vi "Main.vi"() -> ()   [LabVIEW 2024]
doc: "This template is for the Queued Message Handler design pattern.\n\nThe Event Handling Loop generates messages based on user interface actions.\n\nThe Message Handling Loop processes messages generated by the Event Handling Loop, or by other messages. The messages are string values, so new messages can be added easily to the Message Cases case structure in the Message Handling Loop. Each message cluster can also provide an optional value for Message Data, which is a variant that can be converted to whatever message-specific data is required."
uses:
  controls/UI Data.ctl
  support/Message Queue/Enqueue Message (Single).vi
  <vilib>/Utility/error.llb/Error Cluster From Error Code.vi
  <vilib>/ErrorRing/Error Ring.xnode
  support/Message Queue/Message Queue.lvlib
  support/User Event - Stop/User Event - Stop.lvlib
panel:
  out "Display <Replace Me>":string
  in  "Do Something Else <Replace Me>":bool
  in  "Do Something <Replace Me>":bool
  in  "Exit":bool
  # "These controls have associated \"Value Changed\" events configured in the Event Structure on the diagram.\n\nReplace them (and reconfigure the Event Structure) with the controls you need for your application."
  # "This template is for the Queued Message Handler design pattern.\n\nSee the block diagram for more information on how to use this template."
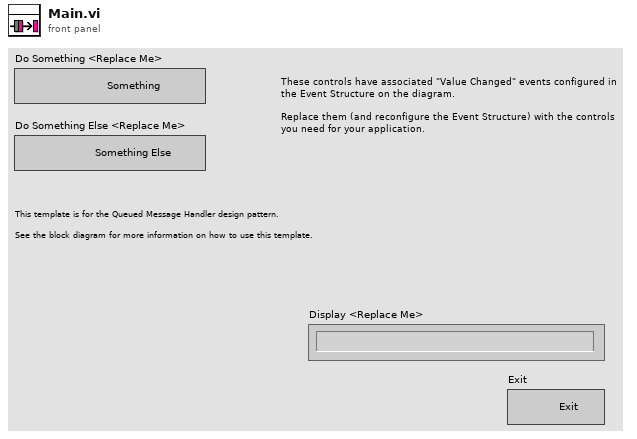
[diagram p1: front panel]
types:
  T1 = typedef "UI Data.ctl" = cluster{"Boolean <Replace Me>":bool, "String <Replace Me>":string, "Numeric <Replace Me>":dbl, "ADK Create MT":refnum<vi>, "ADK Stop":refnum<vi>, "Data Display Ref":refnum<vi>, "Exit Button Ref":refnum<vi>, " ADK Close":refnum<vi>}
  T2 = typedef "Message Queue.lvlib/All Message Queues.ctl" = cluster{"UI":refnum<queue>}
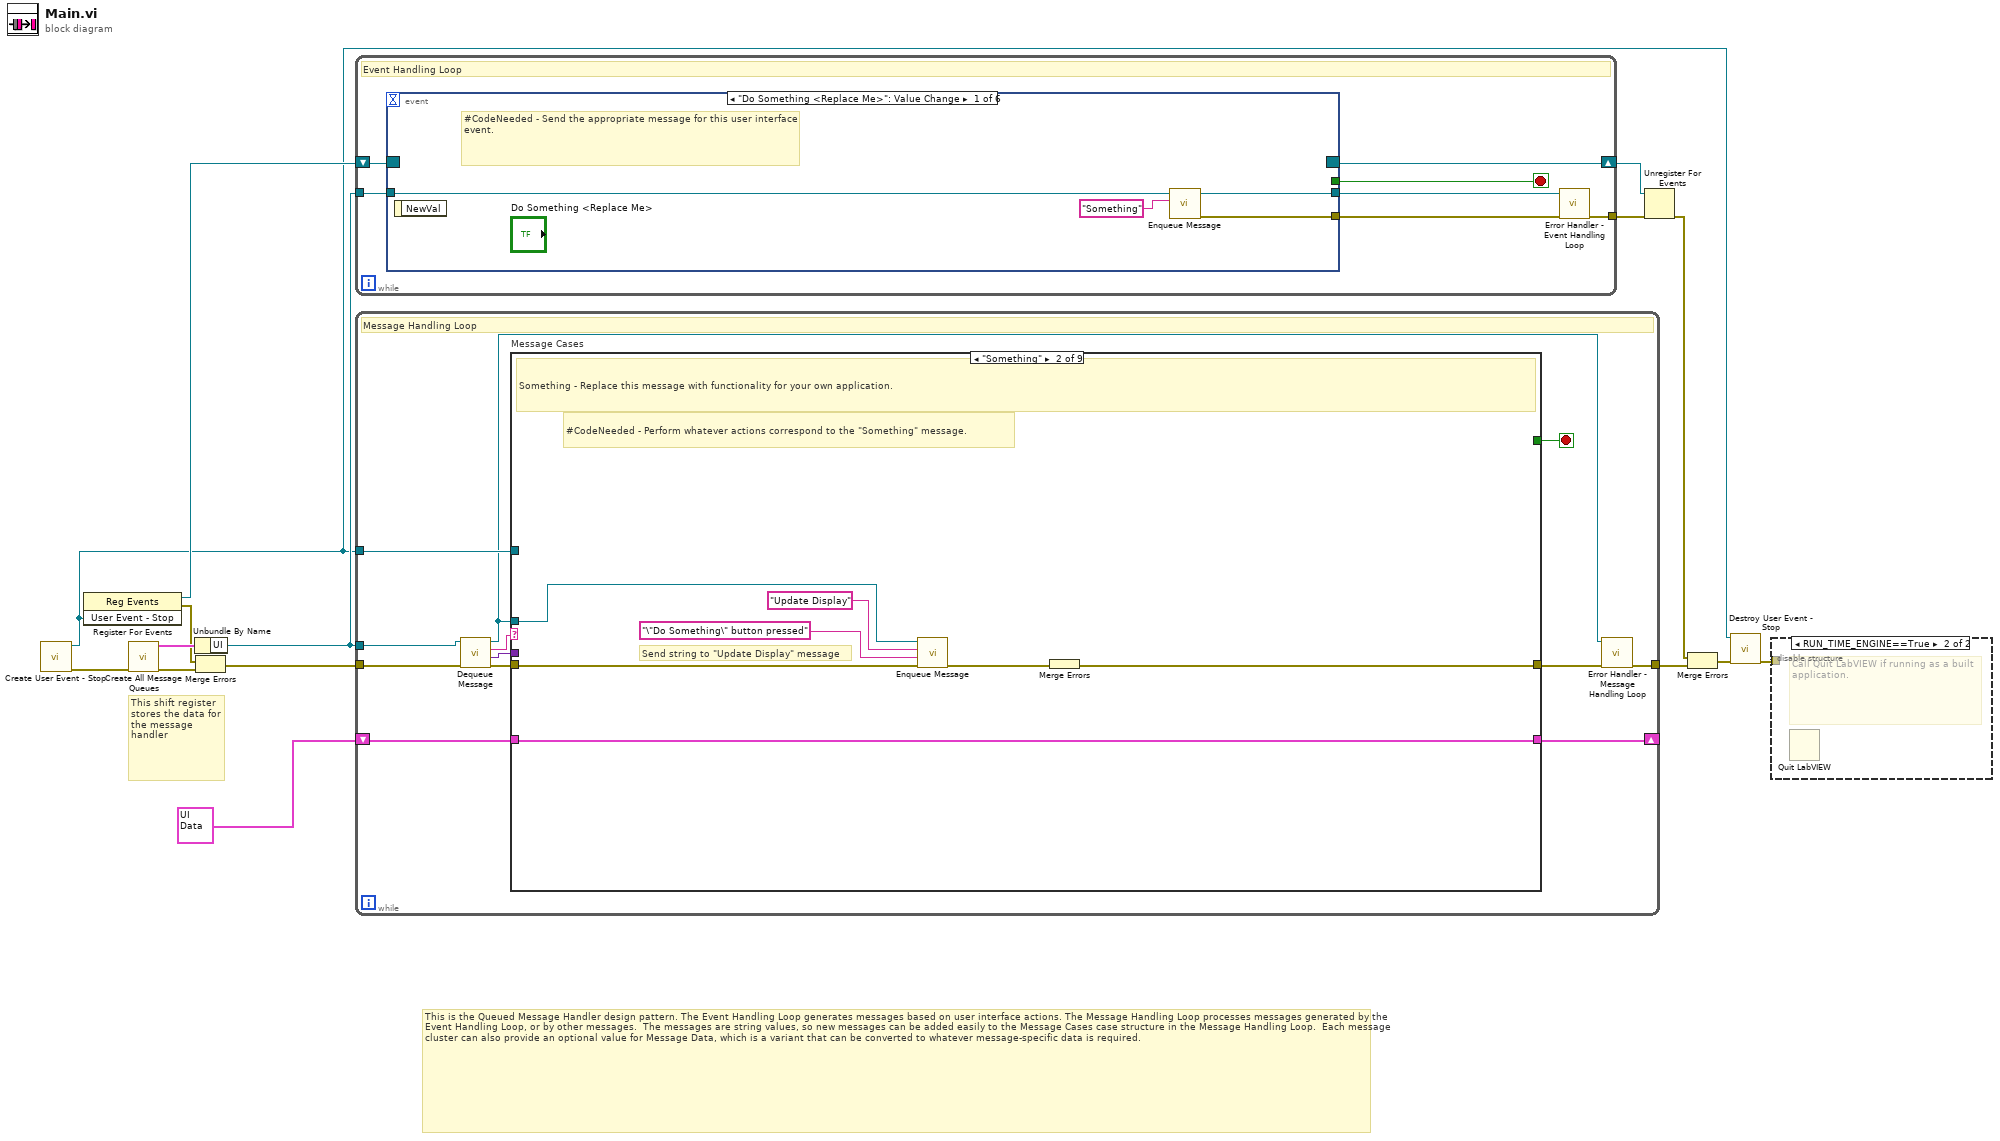
[diagram p0: block diagram]
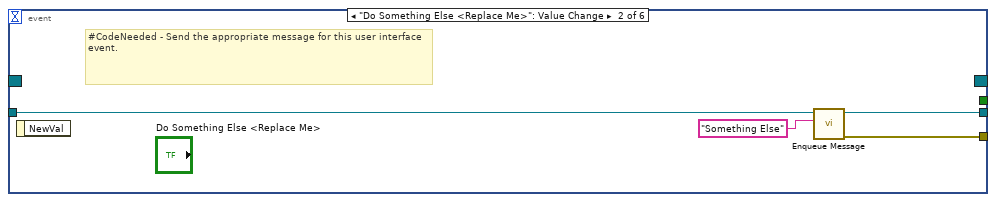
[diagram p3: hidden frame]
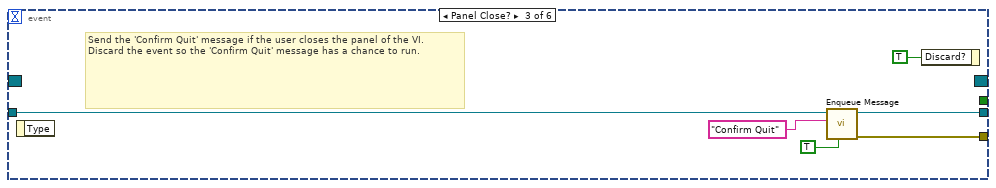
[diagram p4: hidden frame]
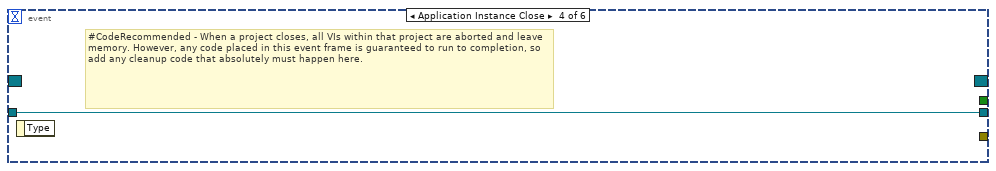
[diagram p5: hidden frame]
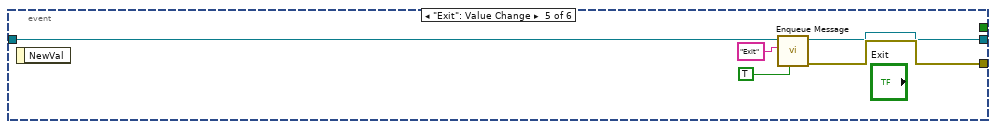
[diagram p6: hidden frame]
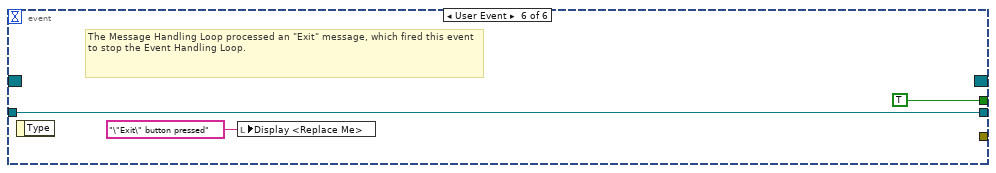
[diagram p7: hidden frame]
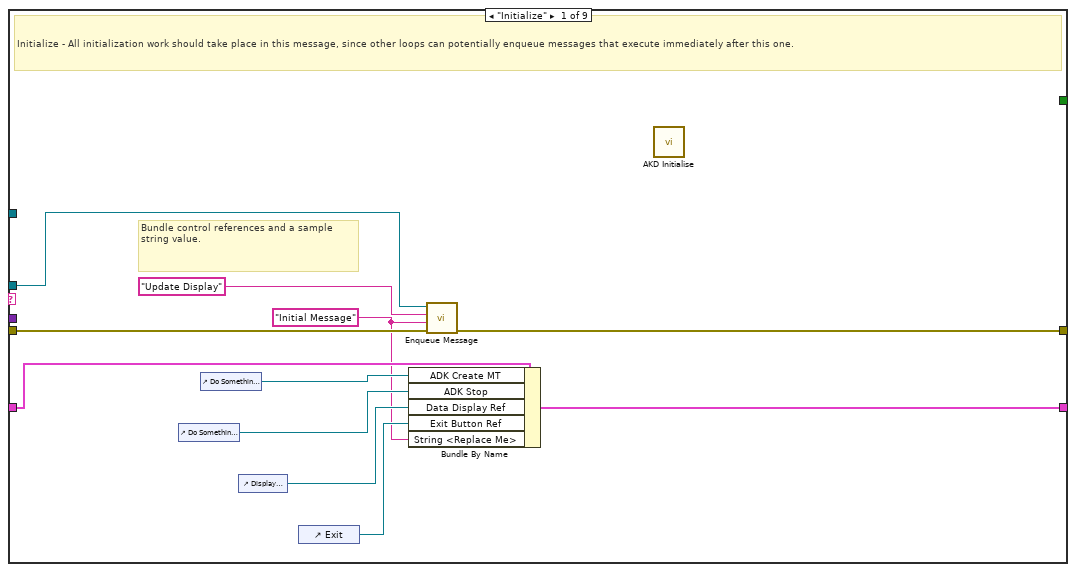
[diagram p8: hidden frame]
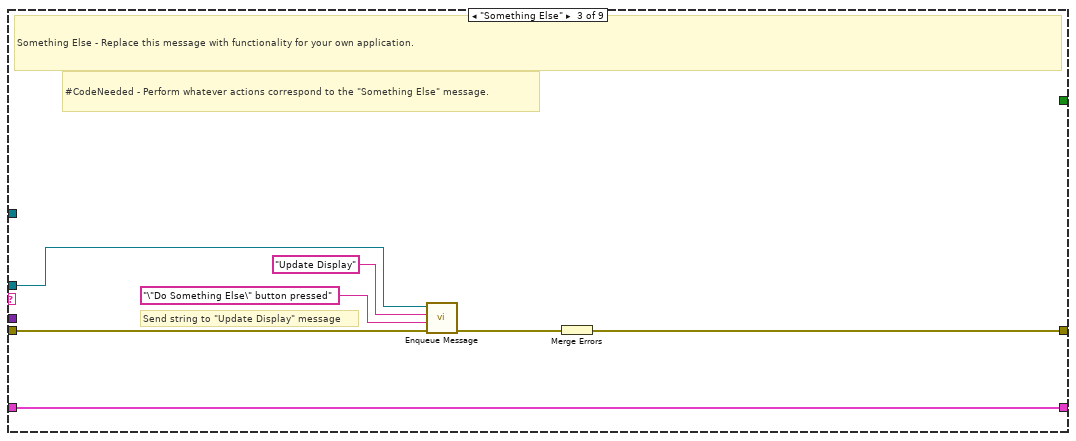
[diagram p9: hidden frame]
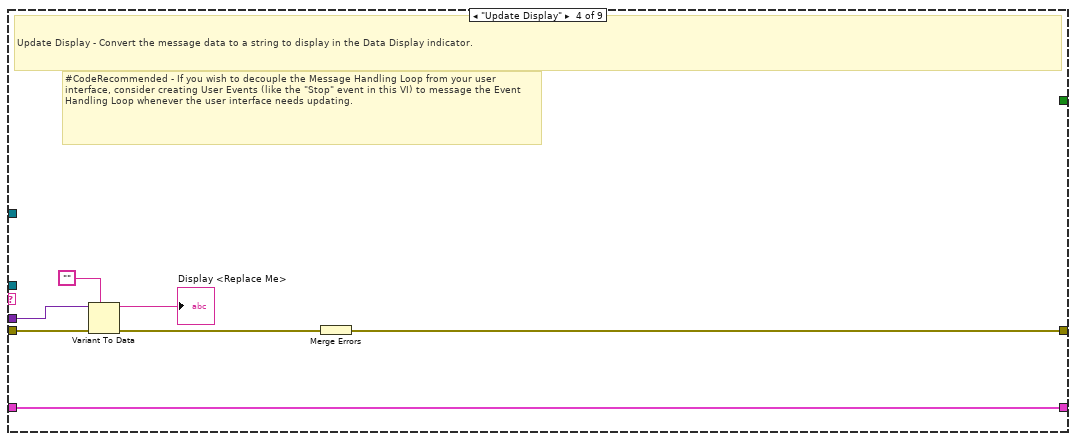
[diagram p10: hidden frame]
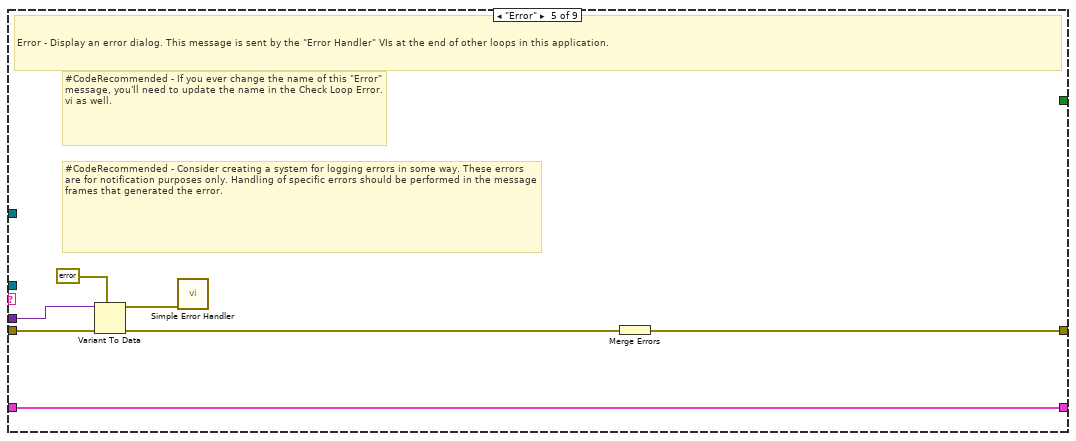
[diagram p11: hidden frame]
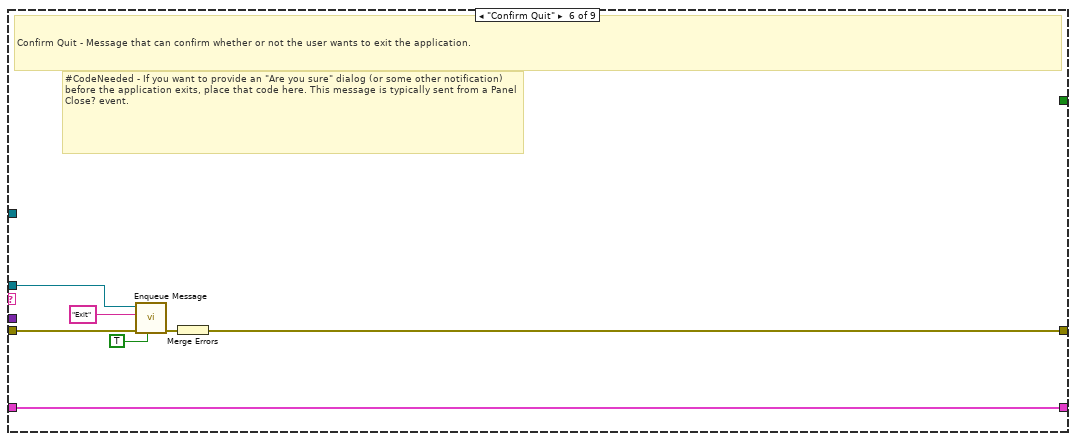
[diagram p12: hidden frame]
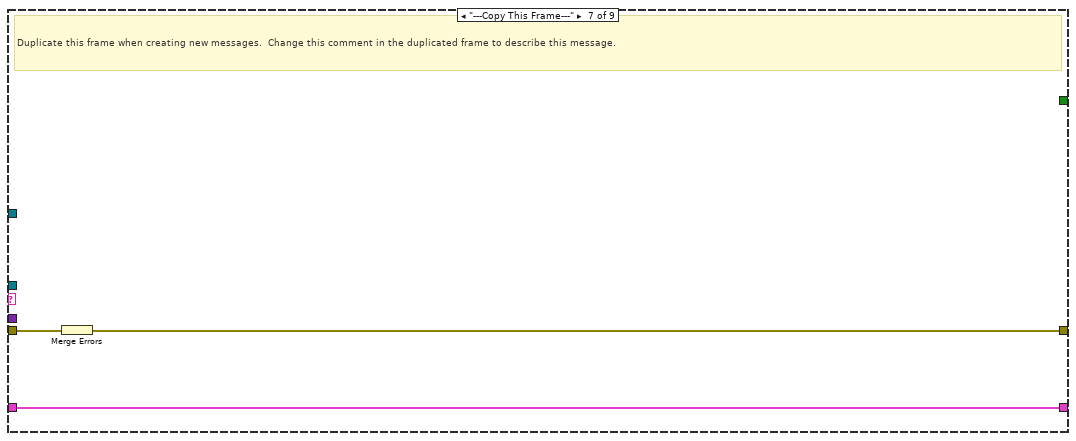
[diagram p13: hidden frame]
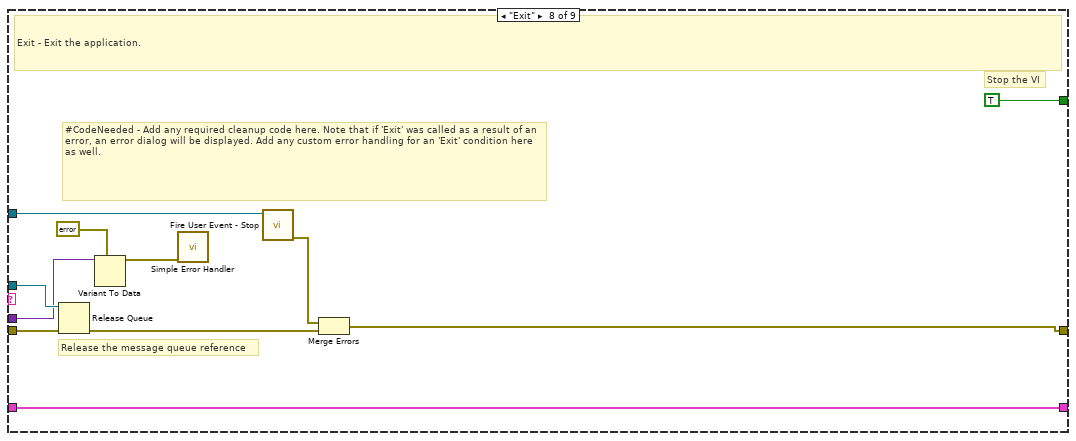
[diagram p14: hidden frame]
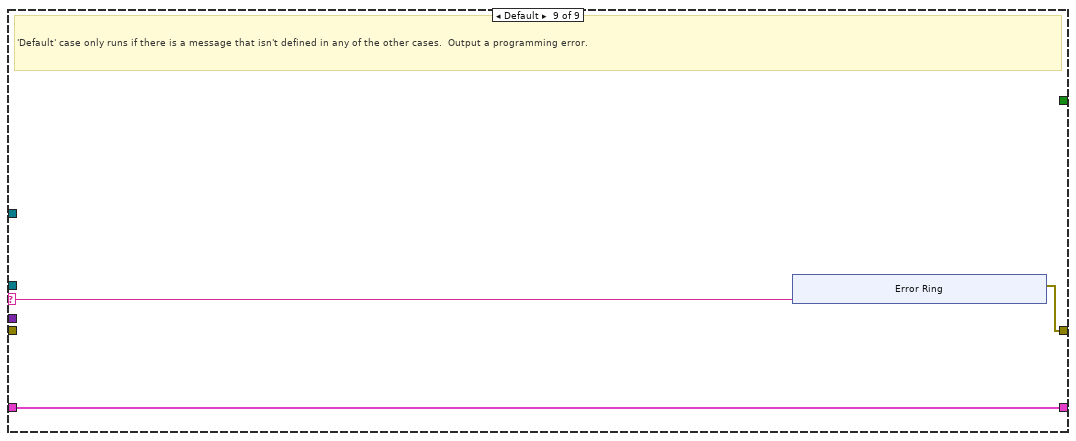
[diagram p15: hidden frame]
diagram:
  # "This is the Queued Message Handler design pattern. The Event Handling Loop generates messages based on user interface actions. The Message Handling Loop processes messages generated by the Event Handling Loop, or by other messages.  The messages are string values, so new messages can be added easily to the Message Cases case structure in the Message Handling Loop.  Each message cluster can also provide an optional value for Message Data, which is a variant that can be converted to whatever message-specific data is required."
  # "This shift register stores the data for the message handler"
  n1 = call "Create User Event - Stop.vi"() -> ("error out"=w11:errorcluster, "User Event - Stop"=w3:refnum<user-event>)  [unwired: 10 in]
  n2 = register-events(w3) -> (reference out=w4:refnum<event-registration>, error out=w1:errorcluster)  [unwired: 2 in]
  n3 = call "Create All Message Queues.vi"("error in (no error)"=w11) -> ("error out"=w15:errorcluster, "Message Queues out"=w14:T2)  [unwired: 9 in]
  n4 = Unbundle By Name(w14) -> ("UI"=w12:refnum<queue>)
  n5 = Merge Errors(w1, w15) -> (w2:errorcluster)
  n6 = while {
    tunnel: w12 -> [w22]
    shift-right: [w20] -> w8
    shift-left: w4 -> [w21]
    tunnel: [w16] -> w5
    stop <- w18 stop-if-true
    # "Event Handling Loop"
    n7 = event shown="[0] \"Do Something <Replace Me>\": Value Change" {
      selector: w21 -> [_ _ _ _ _ _]
      dyn-events: [_ _ _ _ _ _] -> w20
      timeout: _ -> [_ _ _ _ _ _]
      tunnel: [_ _ _ _ _ TRUE ("Discard?")] -> w18
      tunnel: w22 -> [w26 w30 w35 w37 w42 w45]
      tunnel: [w23 w27 w34 _ w41 _] -> w19
      tunnel: [w25 w29 w33 w37 w40 w45] -> w17
      event "Do Something <Replace Me>": Value Change {
        # "#CodeNeeded - Send the appropriate message for this user interface event."
        n8 = event-data() -> ()  [unwired: 1 in, 1 out]
        n9 = call-poly "Enqueue Message.vi"("Message"="Something", "Message Queue"=w26) -> ("error out"=w23:errorcluster, "dup Message Queue"=w25:refnum<queue>)  [unwired: 8 in]
      }
      event "Do Something Else <Replace Me>": Value Change {
        # "#CodeNeeded - Send the appropriate message for this user interface event."
        n10 = event-data() -> ()  [unwired: 1 in, 1 out]
        n11 = call-poly "Enqueue Message.vi"("Message"="Something Else", "Message Queue"=w30) -> ("error out"=w27:errorcluster, "dup Message Queue"=w29:refnum<queue>)  [unwired: 8 in]
      }
      event Panel Close? {
        # "Send the 'Confirm Quit' message if the user closes the panel of the VI. Discard the event so the 'Confirm Quit' message has a chance to run."
        n12 = event-data() -> ()  [unwired: 1 in, 1 out]
        n13 = call-poly "Enqueue Message.vi"("Priority Message? (F)"=TRUE, "Message"="Confirm Quit", "Message Queue"=w35) -> ("error out"=w34:errorcluster, "dup Message Queue"=w33:refnum<queue>)  [unwired: 7 in]
        n14 = event-data("Discard?"=TRUE) -> ()  [unwired: 1 in, 1 out]
      }
      event Application Instance Close {
        # "#CodeRecommended - When a project closes, all VIs within that project are aborted and leave memory. However, any code placed in this event frame is guaranteed to run to completion, so add any cleanup code that absolutely must happen here."
        n15 = event-data() -> ()  [unwired: 1 in, 1 out]
      }
      event "Exit": Value Change {
        n16 = event-data() -> ()  [unwired: 1 in, 1 out]
        n17 = call-poly "Enqueue Message.vi"("Priority Message? (F)"=TRUE, "Message"="Exit", "Message Queue"=w42) -> ("error out"=w41:errorcluster, "dup Message Queue"=w40:refnum<queue>)  [unwired: 7 in]
      }
      event User Event {
        # "The Message Handling Loop processed an \"Exit\" message, which fired this event to stop the Event Handling Loop."
        n18 = event-data() -> ()  [unwired: 1 in, 1 out]
        n19 = local write "Display <Replace Me>"("\"Exit\" button pressed" ("VI Stopped")) -> ()
      }
    }
    n20 = call "Error Handler - Event Handling Loop.vi"("error in (no error)"=w19, "Message Queue"=w17) -> ("dup error in"=w16:errorcluster)  [unwired: 8 in, 1 out]
  }
  n21 = while {
    tunnel: w12 -> [w49]
    shift-right: [w56] -> _
    shift-left: T1 {"Boolean <Replace Me>"=FALSE, "String <Replace Me>"="", "Numeric <Replace Me>"=0.0, "ADK Create MT"=refnum, "ADK Stop"=refnum, "Data Display Ref"=refnum, "Exit Button Ref"=refnum, " ADK Close"=refnum} ("Data Cluster") -> [w57]
    tunnel: w3 -> [w54]
    tunnel: w2 -> [w53]
    tunnel: [w47] -> w13
    stop <- w55 stop-if-true
    # "Message Handling Loop"
    n22 = call "Dequeue Message.vi"("error in (no error)"=w53, "Message Queue"=w49) -> ("error out"=w52:errorcluster, "Message Data"=w50:variant, "Message"=w51:string, "dup Message Queue"=w48:refnum<queue>)  [unwired: 6 in]
    n23 = case "Message Cases" shown="\"Something\"" w51 {
      selector: w51 -> [_ _ _ _ _ _ _ _ w118]
      tunnel: w48 -> [w59 w71 w78 _ _ w99 _ w117 _]
      tunnel: w52 -> [w67 w73 w80 w87 w96 w103 w106 w110 _]
      tunnel: [w68 w74 w81 w88 w90 w101 w104 w113 w119] -> w46
      tunnel: w57 -> [w66 w75 w82 w89 w95 w102 w105 w116 w120]
      tunnel: [w65 w75 w82 w89 w95 w102 w105 w116 w120] -> w56
      tunnel: [_ _ _ _ _ _ _ TRUE _] -> w55
      tunnel: w50 -> [_ _ _ w86 w94 _ _ w107 _]
      tunnel: w54 -> [_ _ _ _ _ _ _ w112 _]
      frame "Initialize" {
        w58 = "Initial Message" ("Initial Message")
        # "Bundle control references and a sample string value."
        # "Initialize - All initialization work should take place in this message, since other loops can potentially enqueue messages that execute immediately after this one."
        n24 = control-ref of="Do Something Else <Replace Me>"() -> (w63:refnum<vi>)
        n25 = control-ref of="Do Something <Replace Me>"() -> (w64:refnum<vi>)
        n26 = control-ref of="Display <Replace Me>"() -> (w62:refnum<vi>)
        n27 = control-ref of="Exit"() -> (w61:refnum<vi>)
        n28 = Bundle By Name(cluster=w66, "ADK Create MT"=w64, "ADK Stop"=w63, "Data Display Ref"=w62, "Exit Button Ref"=w61, "String <Replace Me>"=w58) -> (w65:T1)
        n29 = call-poly "Enqueue Message.vi"("error in (no error)"=w67, "Message Data"=w58, "Message"="Update Display", "Message Queue"=w59) -> ("error out"=w68:errorcluster)  [unwired: 6 in, 1 out]
        n30 = call "AKD Initialise.vi"() -> ()  [unwired: 14 in, 2 out]
      }
      frame "Something" {
        # "Send string to \"Update Display\" message"
        # "#CodeNeeded - Perform whatever actions correspond to the \"Something\" message."
        # "Something - Replace this message with functionality for your own application."
        n31 = call-poly "Enqueue Message.vi"("error in (no error)"=w73, "Message Data"="\"Do Something\" button pressed" ("\"Do Something\" button pressed"), "Message"="Update Display", "Message Queue"=w71) -> ("error out"=w72:errorcluster)  [unwired: 6 in, 1 out]
        n32 = Merge Errors(w72) -> (w74:errorcluster)
      }
      frame "Something Else" {
        # "Send string to \"Update Display\" message"
        # "#CodeNeeded - Perform whatever actions correspond to the \"Something Else\" message."
        # "Something Else - Replace this message with functionality for your own application."
        n33 = call-poly "Enqueue Message.vi"("error in (no error)"=w80, "Message Data"="\"Do Something Else\" button pressed" ("\"Do Something Else\" button pressed"), "Message"="Update Display", "Message Queue"=w78) -> ("error out"=w79:errorcluster)  [unwired: 6 in, 1 out]
        n34 = Merge Errors(w79) -> (w81:errorcluster)
      }
      frame "Update Display" {
        # "#CodeRecommended - If you wish to decouple the Message Handling Loop from your user interface, consider creating User Events (like the \"Stop\" event in this VI) to message the Event Handling Loop whenever the user interface needs updating."
        # "Update Display - Convert the message data to a string to display in the Data Display indicator."
        n35 = Variant To Data(error in=w87, type="", Variant=w86) -> (data=→"Display <Replace Me>":string, error out=w84:errorcluster)
        n36 = Merge Errors(w84) -> (w88:errorcluster)
      }
      frame "Error" {
        # "#CodeRecommended - If you ever change the name of this \"Error\" message, you'll need to update the name in the Check Loop Error.vi as well."
        # "#CodeRecommended - Consider creating a system for logging errors in some way. These errors are for notification purposes only. Handling of specific errors should be performed in the message frames that generated the error."
        # "Error - Display an error dialog. This message is sent by the \"Error Handler\" VIs at the end of other loops in this application."
        n37 = Variant To Data(error in=w96, type=errorcluster {"status"=FALSE, "code"=0, "source"=""} ("error constant"), Variant=w94) -> (data=w92:errorcluster, error out=w91:errorcluster)
        n38 = call <vilib>:"Simple Error Handler.vi"("error in (no error)"=w92) -> ()  [unwired: 4 in, 5 out]
        n39 = Merge Errors(w91) -> (w90:errorcluster)
      }
      frame "Confirm Quit" {
        # "#CodeNeeded - If you want to provide an \"Are you sure\" dialog (or some other notification) before the application exits, place that code here. This message is typically sent from a Panel Close? event."
        # "Confirm Quit - Message that can confirm whether or not the user wants to exit the application."
        n40 = call-poly "Enqueue Message.vi"("Priority Message? (F)"=TRUE, "error in (no error)"=w103, "Message"="Exit", "Message Queue"=w99) -> ("error out"=w100:errorcluster)  [unwired: 6 in, 1 out]
        n41 = Merge Errors(w100) -> (w101:errorcluster)
      }
      frame "---Copy This Frame---" {
        # "Duplicate this frame when creating new messages.  Change this comment in the duplicated frame to describe this message."
        n42 = Merge Errors(w106) -> (w104:errorcluster)
      }
      frame "Exit" {
        # "Stop the VI"
        # "Release the message queue reference"
        # "#CodeNeeded - Add any required cleanup code here. Note that if 'Exit' was called as a result of an error, an error dialog will be displayed. Add any custom error handling for an 'Exit' condition here as well."
        # "Exit - Exit the application."
        n43 = Release Queue(queue=w117, error in (no error)=w110) -> (error out=w114:errorcluster)  [unwired: 1 in, 2 out]
        n44 = Variant To Data(type=errorcluster {"status"=FALSE, "code"=0, "source"=""} ("error constant"), Variant=w107) -> (data=w108:errorcluster)  [unwired: 1 in, 1 out]
        n45 = call <vilib>:"Simple Error Handler.vi"("error in (no error)"=w108) -> ()  [unwired: 4 in, 5 out]
        n46 = call "Fire User Event - Stop.vi"("User Event - Stop"=w112) -> ("error out"=w111:errorcluster)  [unwired: 10 in]
        n47 = Merge Errors(w111, w114) -> (w113:errorcluster)
      }
      frame Default {
        # "'Default' case only runs if there is a message that isn't defined in any of the other cases.  Output a programming error."
        n48 = xnode "Error Ring"("parameter 0"=w118) -> ("error out"=w119:errorcluster)
      }
    }
    n49 = call "Error Handler - Message Handling Loop.vi"("error in (no error)"=w46, "Message Queue"=w48) -> ("dup error in"=w47:errorcluster)  [unwired: 8 in, 1 out]
  }
  n50 = Unregister For Events(event registration refnum=w8, error in=w5) -> (error out=w9:errorcluster)
  n51 = Merge Errors(w9, w13) -> (w10:errorcluster)
  n52 = call "Destroy User Event - Stop.vi"("error in (no error)"=w10, "User Event - Stop"=w3) -> ("error out"=w6:errorcluster)  [unwired: 9 in]
  n53 = disable-structure shown="RUN_TIME_ENGINE==True" {
    disable-tunnel: w6 -> [_ _]
    frame condition #0 (active) {
    }
    frame condition #1 {
      # "Call Quit LabVIEW if running as a built application."
      n54 = Quit LabVIEW() -> ()  [unwired: 1 in]
    }
  }
